vi "S4ICS Batch-Extract.vi"() -> ()   [LabVIEW 2018]
uses:
  <vilib>/Analysis/NI_AALBase.lvlib
panel:
  out "size(#)":i32
  out "Min":i32
  out "Max":i32
  out "Histogram Graph":T1(graph)
  out "variance":dbl format="%0.2f"
  out "std dev":dbl format="%0.2f"
  out "mean":dbl format="%0.2f"
  out "cmd #":i32
  out "current time":timestamp format="%<%H:%M:%S%3u\n%Y/%m/%d>T"
  out "batch cmd":string
  in  "batch file":string="WPROT" caption="Batch File Name"
  in  "allin":T2={"s4icsIP"="localhost", "s4icsPort"=54165, "mech name"="", "cmd"=[], "log"=refnum} {"s4icsPort" min=1025 step=1}
  in  "stop":bool
  # "S4ICS Batch - Extract LTE"
  # "Extracted LaTched Encoder Positions"
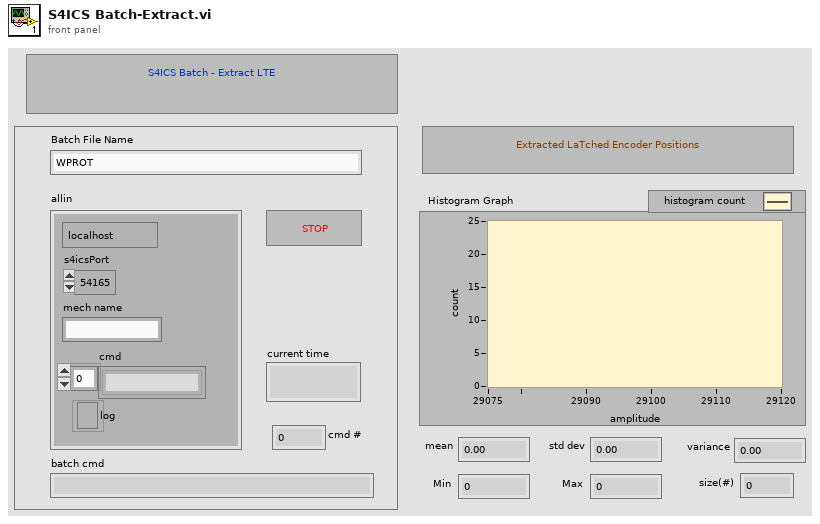
[diagram p1: front panel]
types:
  T1 = cluster{"X Values":dbl[], "Histogram: h(x)":i32[]}
  T2 = cluster{"s4icsIP":string, "s4icsPort":u16, "mech name":string, "cmd":string[], "log":refnum<file>}
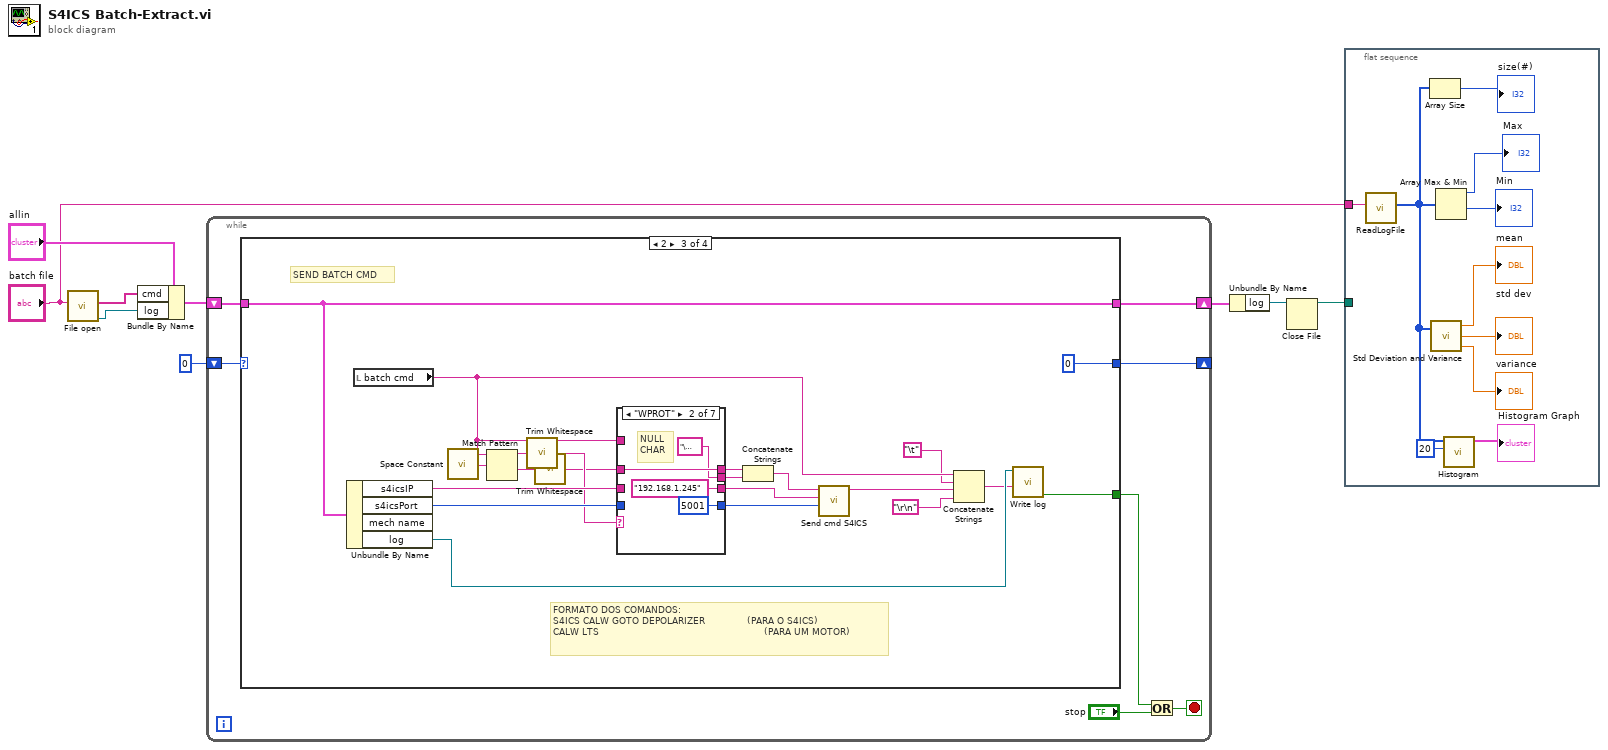
[diagram p0: block diagram]
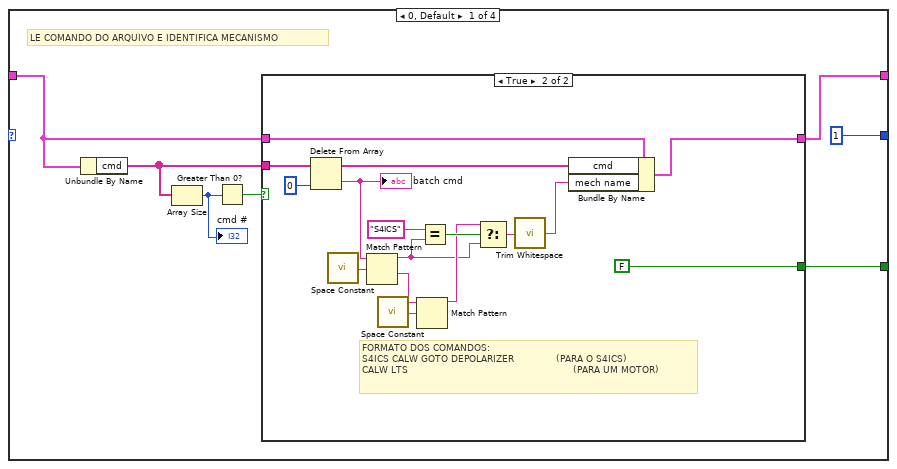
[diagram p2: hidden frame]
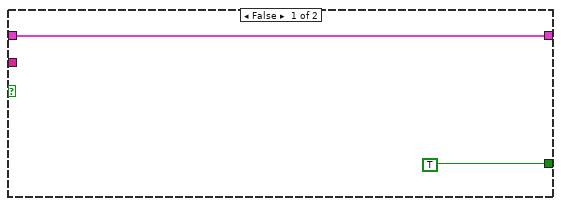
[diagram p3: hidden frame]
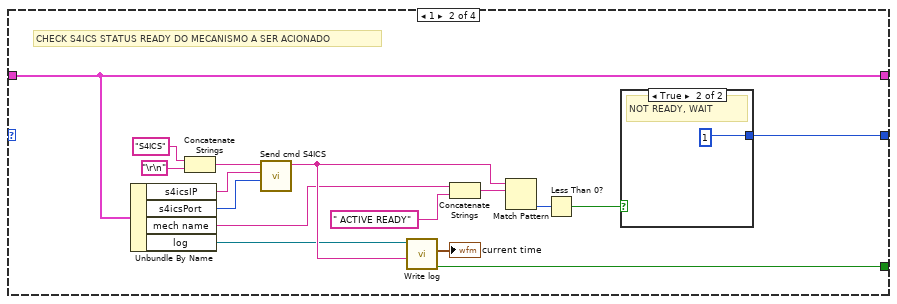
[diagram p4: hidden frame]
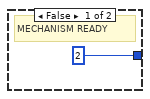
[diagram p5: hidden frame]
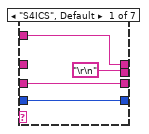
[diagram p6: hidden frame]
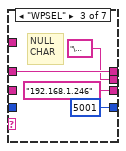
[diagram p7: hidden frame]
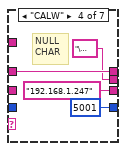
[diagram p8: hidden frame]
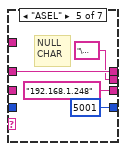
[diagram p9: hidden frame]
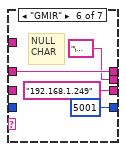
[diagram p10: hidden frame]
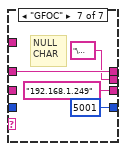
[diagram p11: hidden frame]
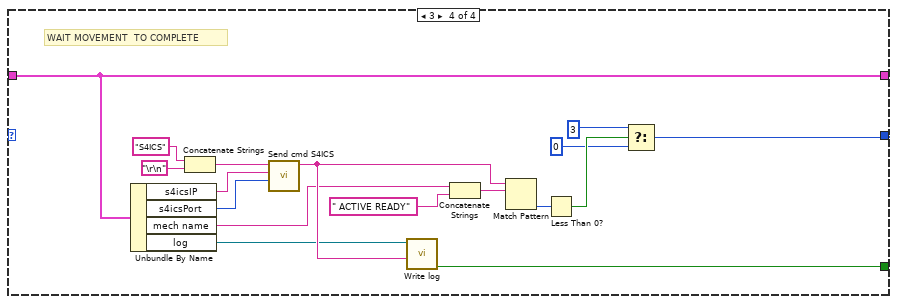
[diagram p12: hidden frame]
diagram:
  n1 = call "File open.vi"("file name"="batch file") -> ("log"=w6:refnum<file>, "cmd"=w5:string[])  [unwired: 9 in]
  n2 = Bundle By Name(cluster="allin", "cmd"=w5, "log"=w6) -> (w7:T2)
  n3 = while {
    shift-right: [w15] -> _
    shift-left: u8 0 -> [w16]
    shift-right: [w13] -> w4
    shift-left: w7 -> [w14]
    stop <- w11 stop-if-true
    n4 = case shown="2" w16 {
      tunnel: [u8 1 ("x+1") w42 u8 0 ("x+1") w124] -> w15
      tunnel: w14 -> [w21 w50 w78 w125]
      tunnel: [w18 w50 w78 w125] -> w13
      tunnel: [w20 w48 w69 w123] -> w10
      frame 0, Default {
        # "LE COMANDO DO ARQUIVO E IDENTIFICA MECANISMO"
        n5 = Unbundle By Name(w21) -> ("cmd"=w17:string[])
        n6 = Array Size(array=w17) -> (size(s)=w23:i32)
        "cmd #" <- w23
        n7 = Greater Than 0?(x=w23) -> (x > 0?=w22:bool)
        n8 = case shown="True" w22 {
          tunnel: w17 -> [_ w41]
          tunnel: w21 -> [w25 w40]
          tunnel: [w25 w39] -> w18
          tunnel: [TRUE FALSE] -> w20
          frame False {
          }
          frame True {
            # "FORMATO DOS COMANDOS:\nS4ICS CALW GOTO DEPOLARIZER              (PARA O S4ICS)\nCALW LTS                                                       (PARA UM MOTOR)"
            n9 = Delete From Array(array=w41, index=0) -> (deleted portion=w35:string, array with subset deleted=w38:string[])  [unwired: 1 in]
            "batch cmd" <- w35
            n10 = call <vilib>:"Space Constant.vi"() -> ("String"=w36:string)
            n11 = Match Pattern(string=w35, regular expression=w36) -> (before substring=w28:string, after substring=w32:string)  [unwired: 1 in, 2 out]
            n12 = call <vilib>:"Space Constant.vi"() -> ("String"=w33:string)
            n13 = Match Pattern(string=w32, regular expression=w33) -> (before substring=w29:string)  [unwired: 1 in, 3 out]
            n14 = Equal?(x="S4ICS", y=w28) -> (x = y?=w30:bool)
            n15 = Select(t=w29, s=w30, f=w28) -> (s? t:f=w27:string)
            n16 = call <vilib>:"Trim Whitespace.vi"("string"=w27) -> ("trimmed string"=w26:string)  [unwired: 1 in]
            n17 = Bundle By Name(cluster=w40, "cmd"=w38, "mech name"=w26) -> (w39:T2)
          }
        }
      }
      frame 1 {
        # "CHECK S4ICS STATUS READY DO MECANISMO A SER ACIONADO"
        n18 = Unbundle By Name(w50) -> ("s4icsIP"=w55:string, "s4icsPort"=w54:u16, "mech name"=w45:string, "log"=w47:refnum<file>)
        n19 = Concatenate Strings("S4ICS", "\r\n") -> (w53:string)
        n20 = call "Send cmd S4ICS.vi"("port"=w54, "address"=w55, "data in"=w53) -> ("data out"=w49:string)  [unwired: 7 in, 1 out]
        n21 = call "Write log.vi"("text"=w49, "log file"=w47) -> ("status"=w48:bool, "current time"=→"current time":timestamp)  [unwired: 8 in]
        n22 = Concatenate Strings(w45, " ACTIVE READY") -> (w46:string)
        n23 = Match Pattern(string=w49, regular expression=w46) -> (offset past match=w52:i32)  [unwired: 1 in, 3 out]
        n24 = Less Than 0?(x=w52) -> (x < 0?=w43:bool)
        n25 = case shown="True" w43 {
          tunnel: [u8 2 ("f") u8 1 ("f")] -> w42
          frame False {
            # "MECHANISM READY"
          }
          frame True {
            # "NOT READY, WAIT"
          }
        }
      }
      frame 2 {
        # "FORMATO DOS COMANDOS:\nS4ICS CALW GOTO DEPOLARIZER              (PARA O S4ICS)\nCALW LTS                                                       (PARA UM MOTOR)"
        # "SEND BATCH CMD"
        n26 = Unbundle By Name(w78) -> ("s4icsIP"=w80:string, "s4icsPort"=w79:u16, "log"=w68:refnum<file>)  [unwired: 1 out]
        n27 = local read "batch cmd"() -> (w67:string)
        n28 = call <vilib>:"Space Constant.vi"() -> ("String"=w73:string)
        n29 = Match Pattern(string=w67, regular expression=w73) -> (before substring=w63:string, after substring=w72:string)  [unwired: 1 in, 2 out]
        n30 = call <vilib>:"Trim Whitespace.vi"("string"=w63) -> ("trimmed string"=w62:string)  [unwired: 1 in]
        n31 = call <vilib>:"Trim Whitespace.vi"("string"=w72) -> ("trimmed string"=w61:string)  [unwired: 1 in]
        n32 = case shown="\"WPROT\"" w62 {
          tunnel: w80 -> [w84 _ _ _ _ _ _]
          tunnel: w79 -> [w83 _ _ _ _ _ _]
          tunnel: [w84 "192.168.1.245" ("s4icsIP") "192.168.1.246" ("s4icsIP") "192.168.1.247" ("s4icsIP") "192.168.1.248" ("s4icsIP") "192.168.1.249" ("s4icsIP") "192.168.1.249" ("s4icsIP")] -> w76
          tunnel: [w83 u16 5001 ("s4icsPort") u16 5001 ("s4icsPort") u16 5001 ("s4icsPort") u16 5001 ("s4icsPort") u16 5001 ("s4icsPort") u16 5001 ("s4icsPort")] -> w75
          tunnel: w61 -> [_ w86 w90 w94 w98 w102 w106]
          tunnel: w67 -> [w82 _ _ _ _ _ _]
          tunnel: [w82 w86 w90 w94 w98 w102 w106] -> w71
          tunnel: ["\r\n" "\u0000" ("search string") "\u0000" ("search string") "\u0000" ("search string") "\u0000" ("search string") "\u0000" ("search string") "\u0000" ("search string")] -> w70
          frame "S4ICS", Default {
          }
          frame "WPROT" {
            # "NULL\nCHAR"
          }
          frame "WPSEL" {
            # "NULL\nCHAR"
          }
          frame "CALW" {
            # "NULL\nCHAR"
          }
          frame "ASEL" {
            # "NULL\nCHAR"
          }
          frame "GMIR" {
            # "NULL\nCHAR"
          }
          frame "GFOC" {
            # "NULL\nCHAR"
          }
        }
        n33 = Concatenate Strings(w71, w70) -> (w74:string)
        n34 = call "Send cmd S4ICS.vi"("port"=w75, "address"=w76, "data in"=w74) -> ("data out"=w66:string)  [unwired: 7 in, 1 out]
        n35 = Concatenate Strings(w67, "\t", w66, "\r\n") -> (w65:string)
        n36 = call "Write log.vi"("text"=w65, "log file"=w68) -> ("status"=w69:bool)  [unwired: 8 in, 1 out]
      }
      frame 3 {
        # "WAIT MOVEMENT  TO COMPLETE"
        n37 = Unbundle By Name(w125) -> ("s4icsIP"=w120:string, "s4icsPort"=w119:u16, "mech name"=w110:string, "log"=w112:refnum<file>)
        n38 = Concatenate Strings("S4ICS", "\r\n") -> (w118:string)
        n39 = call "Send cmd S4ICS.vi"("port"=w119, "address"=w120, "data in"=w118) -> ("data out"=w113:string)  [unwired: 7 in, 1 out]
        n40 = call "Write log.vi"("text"=w113, "log file"=w112) -> ("status"=w123:bool)  [unwired: 8 in, 1 out]
        n41 = Concatenate Strings(w110, " ACTIVE READY") -> (w111:string)
        n42 = Match Pattern(string=w113, regular expression=w111) -> (offset past match=w117:i32)  [unwired: 1 in, 3 out]
        n43 = Less Than 0?(x=w117) -> (x < 0?=w115:bool)
        n44 = Select(t=u8 3 ("f"), s=w115, f=u8 0) -> (s? t:f=w124:u8)
      }
    }
    n45 = Or(x=w10, y="stop") -> (x .or. y?=w11:bool)
  }
  n46 = Unbundle By Name(w4) -> ("log"=w3:refnum<file>)
  n47 = Close File(refnum=w3) -> (path=w1:path)  [unwired: 1 in, 1 out]
  n48 = flat-sequence {
    tunnel: "batch file" -> [w135]
    tunnel: w1 -> [_]
    frame #0 {
      n49 = call "ReadLogFile.vi"("file name"=w135) -> ("Array"=w127:i32[])  [unwired: 10 in]
      n50 = Array Size(array=w127) -> (size(s)=→"size(#)":i32)
      n51 = call <vilib>:"Std Deviation and Variance.vi"("X"=w127) -> ("mean"=→"mean":dbl, "standard deviation"=→"std dev":dbl, "variance"=→"variance":dbl)  [unwired: 1 in]
      n52 = Array Max & Min(array=w127) -> (max value=→"Max":i32, min value=→"Min":i32)  [unwired: 2 out]
      n53 = call <vilib>:"Histogram.vi"("intervals"=20, "X"=w127) -> ("Histogram Graph"=→"Histogram Graph":T1)  [unwired: 6 in, 3 out]
    }
  }
